vi "Utility Generate Instrument Error.vi"(7 "Message":string, 8 "error in (no error)":errorcluster {"code" format="%.0x"}, 9 "Code (0)":i32 format="%.0x", 10 "Is Warning? (F)":bool, 11 "VISA session":refnum<visa-resource-name>) -> (0 "error out":errorcluster {"code" format="%.0x"}, 3 "dup VISA session":refnum<visa-resource-name>)   [LabVIEW 2011]
doc: "Builds the Error Out cluster using input information. Status is set to true if Is warning? is set to FALSE. Code in the Error Out cluster is set to the value in Code. Source appends Message to the chain of callers fromt he VI that produced the error or warning. The VI chain information does not include the name of this VI.\n\nNote: If an error occurred before this VI runs, the VI passes the error in value to Error Out. The Error Out is not modifed by this VI."
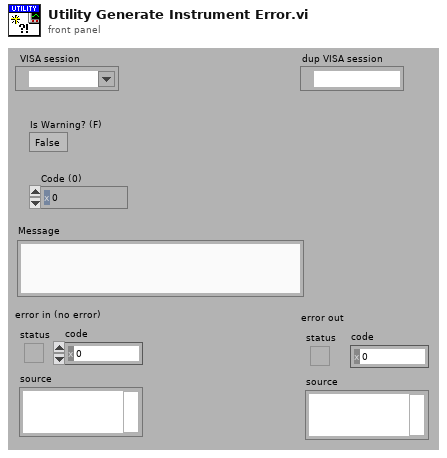
[diagram p1: front panel]
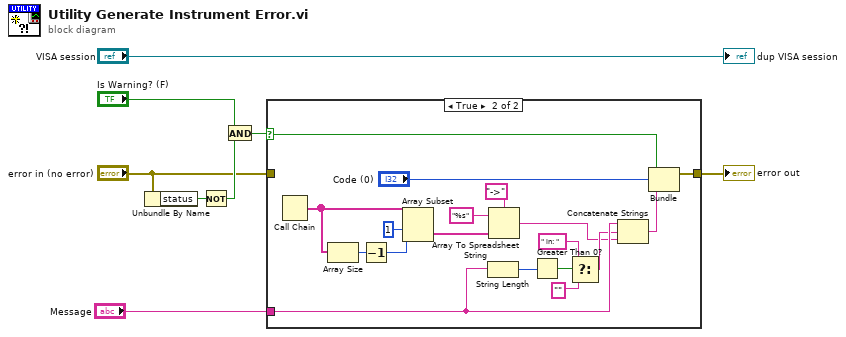
[diagram p0: block diagram]
diagram:
  n1 = Unbundle By Name("error in (no error)") -> ("status"=w8:bool)
  n2 = Not(x=w8) -> (.not. x?=w6:bool)
  n3 = And(x="Is Warning? (F)", y=w6) -> (x .and. y?=w4:bool)
  n4 = case shown="True" w4 {
    selector: w4 -> [_ w19]
    tunnel: [w9 w20] -> w7
    tunnel: "error in (no error)" -> [w9 _]
    tunnel: "Message" -> [_ w12]
    frame False {
    }
    frame True {
      n5 = Call Chain() -> (call chain=w26:string[])
      n6 = Array Size(array=w26) -> (size(s)=w25:i32)
      n7 = Decrement(x=w25) -> (x-1=w24:i32)
      n8 = Array Subset(array=w26, index=1 ("Array Index"), length=w24) -> (w18:string[])
      n9 = String Length(string=w12) -> (length=w16:i32)
      n10 = Array To Spreadsheet String(delimiter (Tab)="->", array=w18, 3:"%s" ("format string")) -> (spreadsheet string=w10:string)
      n11 = Greater Than 0?(x=w16) -> (x > 0?=w15:bool)
      n12 = Select(t=" in: " ("string"), s=w15, f="" ("string")) -> (s? t:f=w11:string)
      n13 = Concatenate Strings(w12, w11, w10) -> (w17:string)
      n14 = Bundle(w19, "Code (0)"="Code (0)", w17) -> (w20:cluster{bool, "Code (0)":i32, string})  [unwired: 1 in]
    }
  }
  "error out" <- w7
  "dup VISA session" <- "VISA session"
